vi "Remove Current Tab.vi"(8 "error in (no error)":errorcluster, 11 "CIF_UI in":refnum<class "CIF_UI.lvclass">) -> (0 "error out":errorcluster)   [LabVIEW 2021, in "CIF_UI.lvclass"]
uses:
  CIF_UI.lvclass
  CIF_UI.lvclass/CIF_UI.ctl
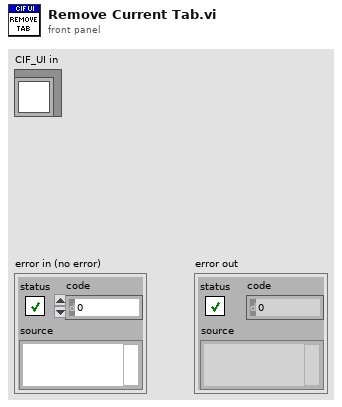
[diagram p1: front panel]
types:
  T1 = typedef "CIF_Manager_UI_Tab.ctl" = enum32{"System Management", "Channels", "Monitoring and Errors", "Plugin", "Plugin2", "Plugin3", "Plugin4", "Plugin5", "Plugin6", "Plugin7", "Plugin8", "Plugin9", "Plugin10"}
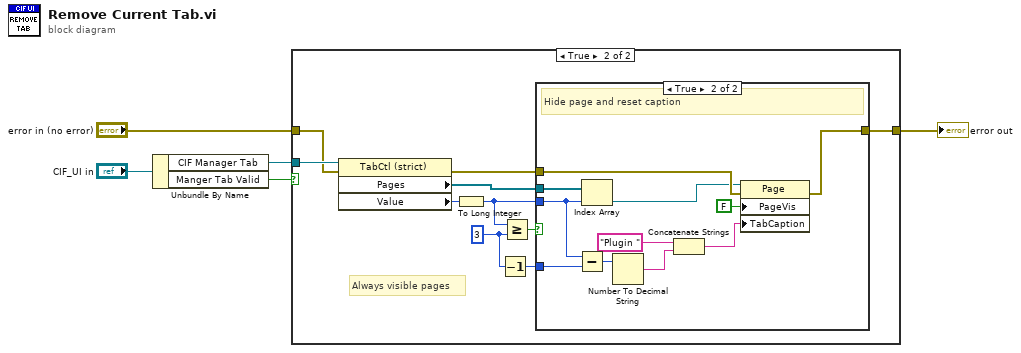
[diagram p0: block diagram]
diagram:
  n1 = Unbundle By Name("CIF_UI in") -> ("CIF Manager Tab"=w3:refnum<vi>, "Manger Tab Valid"=w4:bool)
  n2 = case shown="True" w4 {
    tunnel: w3 -> [_ w16]
    tunnel: "error in (no error)" -> [w6 w14]
    tunnel: [w6 w13] -> w1
    frame False {
    }
    frame True {
      w7 = 3 ("y")
      # "Always visible pages"
      n3 = property class="TabCtl (strict)"(reference=w16, error in=w14) -> (error out=w15:errorcluster, "Pages"=w12:refnum<vi>[], "Value"=w11:T1)  [unwired: 1 out]
      n4 = To Long Integer(number=w11) -> (32bit integer=w10:i32)
      n5 = Decrement(x=w7) -> (x-1=w8:i32)
      n6 = Greater Or Equal?(x=w10, y=w7) -> (x >= y?=w9:bool)
      n7 = case shown="True" w9 {
        tunnel: w15 -> [w17 w28]
        tunnel: [w17 w18] -> w13
        tunnel: w12 -> [_ w27]
        tunnel: w10 -> [_ w22]
        tunnel: w8 -> [_ w20]
        frame False {
          # "Can't hide first two tabs"
        }
        frame True {
          # "Hide page and reset caption"
          n8 = Subtract(x=w22, y=w20) -> (x-y=w21:i32)
          n9 = Index Array(array=w27, index=w22) -> (element=w26:refnum<vi>)
          n10 = Number To Decimal String(number=w21) -> (decimal integer string=w25:string)  [unwired: 1 in]
          n11 = Concatenate Strings("Plugin " ("string"), w25) -> (w19:string)
          n12 = property class="Page"(reference=w26, error in=w28, "PageVis"=FALSE ("Page Visible"), "TabCaption"=w19) -> (error out=w18:errorcluster)  [unwired: 1 out]
        }
      }
    }
  }
  "error out" <- w1
